vi "Main.vi"() -> ()   [LabVIEW 2014, in "DB_CONNECTOR.lvlib"]
doc: "Database Connector DQMH module. \n\nThis module is a singleton. Every module or component within an application that needs database connectivity should load its own instance of this module and keep the reference private.\n\n_____\nBased on Delacor QMH Project Template 4.0.0.43.\n\n<b>Note:</b> This VI was modified by the <b>Validate DQMH Module</b> tool to upgrade it to the DQMH 5.0 approach to destroying cloneable module event references.\n\n<b>Note:</b> This VI was modified by the <b>Validate DQMH Module</b> tool to have the module name be passed as the Additional Information parameter with an Error Reported broadcast.\n\n<b>Note:</b> This VI was modified by the <b>Validate DQMH Module</b> tool to call the Release Message Queue VI in the top-level Error case."
uses:
  DB_CONNECTOR.lvlib
  <vilib>/Delacor/Delacor QMH/Libraries/Cloneable Module Admin_class/Delacor_lib_QMH_Cloneable Module Admin.lvclass
  Module Data--cluster.ctl
  DB-Interface/DB-Interface.lvclass
  DB-Interface/DB-MySQL/Network Config.ctl
  <vilib>/Delacor/Delacor QMH/Libraries/Message Queue_class/Delacor_lib_QMH_Message Queue.lvclass/Delacor_lib_QMH_Message Queue.ctl
  <vilib>/Delacor/Delacor QMH/Libraries/Cloneable Module Admin_class/Delacor_lib_QMH_Cloneable Module Admin.lvclass/Delacor_lib_QMH_Cloneable Module Admin.ctl
  Stop Argument--cluster.ctl
  <vilib>/Delacor/Delacor QMH/Libraries/Module Admin_class/Delacor_lib_QMH_Module Admin.lvclass/Delacor_lib_QMH_Module Admin.ctl
  Configure Argument--cluster.ctl
  Connect Argument--cluster.ctl
  Query Argument--cluster.ctl
  Query (Reply Payload)--cluster.ctl
  Fast Query Argument--cluster.ctl
  Close Connection Argument--cluster.ctl
  Start Transaction Argument--cluster.ctl
  Commit Transaction Argument--cluster.ctl
  Commit Transaction (Reply Payload)--cluster.ctl
  Get DB-Type Argument--cluster.ctl
  Get DB-Type (Reply Payload)--cluster.ctl
  <vilib>/Utility/miscctls.llb/LVPointTypeDef.ctl
  <vilib>/Delacor/Delacor QMH/Libraries/Message Queue_class/Delacor_lib_QMH_Enqueue Message (Single).vi
  <vilib>/Delacor/Delacor QMH/Libraries/Cloneable Module Admin_class/Delacor_lib_QMH_Get Module ID.vi
  <vilib>/Delacor/Delacor QMH/Libraries/Module Admin_class/Delacor_lib_QMH_Get External Launch.vi
  <vilib>/Utility/error.llb/Error Cluster From Error Code.vi
  <vilib>/ErrorRing/Error Ring.xnode
  <vilib>/Delacor/Delacor QMH/Libraries/Message Queue_class/Delacor_lib_QMH_Message Queue.lvclass
  DB-Interface/DB-MySQL/DB-MySQL.lvclass
panel:
  in  "Config Section":string
  in  "Call Chain":string[](array[string])
  out "Module Name":string
  in  "Simulate MHL Error":bool
  in  "Simulate EHL Error":bool
  out "error out":errorcluster
  in  "Module Admin":refnum<class "Delacor_lib_QMH_Cloneable Module Admin.lvclass">
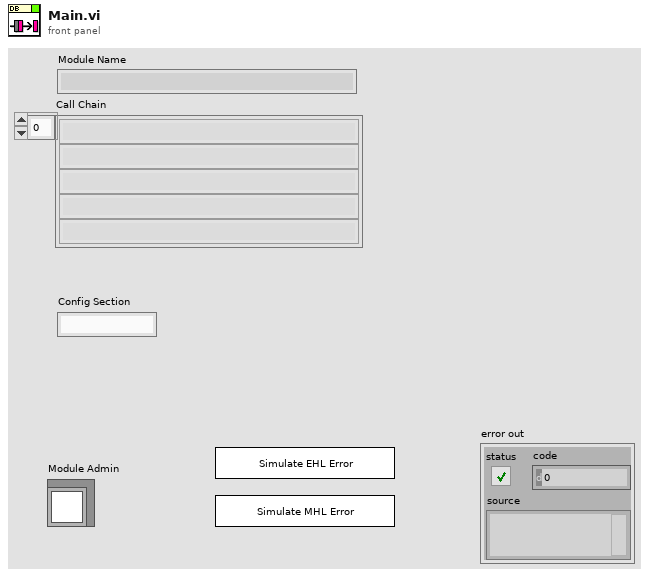
[diagram p1: front panel]
types:
  T1 = typedef "DB_CONNECTOR.lvlib/Request Events--cluster.ctl" = cluster{"Stop Module":refnum<user-event>, "Show Panel":refnum<user-event>, "Hide Panel":refnum<user-event>, "Show Diagram":refnum<user-event>, "Get Module Execution Status":refnum<user-event>, "Configure":refnum<user-event>, "Connect":refnum<user-event>, "Query":refnum<user-event>, "Close Connection":refnum<user-event>, "Start Transaction":refnum<user-event>, "Commit Transaction":refnum<user-event>, "Fast Query":refnum<user-event>, "Get DB-Type":refnum<user-event>}
  T2 = typedef "DB_CONNECTOR.lvlib/Module Data--cluster.ctl" = cluster{"Config Section":string, "DB-Interface":refnum<class "DB-Interface.lvclass">, "Driver":string, "DB-Type":string, "Authentication":cluster{"User":string, "Password":string, "Database":string}, "Network Config":T3}
  T3 = typedef "hse-db.lvlib/DB-MySQL.lvclass/Network Config.ctl" = cluster{"IP Address":string, "Port":u16, "Timeout ms":i32}
  T4 = enum32{"invalid lock state", "Not Locked", "Locked (No Password)", "Password-protected"}
  T5 = typedef "DB_CONNECTOR.lvlib/Stop Argument--cluster.ctl" = cluster{"Origin":string, "Module ID":i32, "Exit via Stop Module Req?":bool, "Wait for Module to stop?":bool}
  T6 = typedef "DB_CONNECTOR.lvlib/Configure Argument--cluster.ctl" = cluster{"Module ID":i32, "Boolean":bool}
  T7 = typedef "DB_CONNECTOR.lvlib/Connect Argument--cluster.ctl" = cluster{"Module ID":i32, "Boolean":bool}
  T8 = typedef "DB_CONNECTOR.lvlib/Query Argument--cluster.ctl" = cluster{"Module ID":i32, "Query":string, "Wait Notifier":refnum<notifier>}
  T9 = typedef "DB_CONNECTOR.lvlib/Fast Query Argument--cluster.ctl" = cluster{"Module ID":i32, "Query":string}
  T10 = typedef "DB_CONNECTOR.lvlib/Close Connection Argument--cluster.ctl" = cluster{"Module ID":i32, "Boolean":bool}
  T11 = typedef "DB_CONNECTOR.lvlib/Start Transaction Argument--cluster.ctl" = cluster{"Module ID":i32, "Boolean":bool}
  T12 = typedef "DB_CONNECTOR.lvlib/Commit Transaction Argument--cluster.ctl" = cluster{"Module ID":i32, "Wait Notifier":refnum<notifier>}
  T13 = typedef "DB_CONNECTOR.lvlib/Get DB-Type Argument--cluster.ctl" = cluster{"Module ID":i32, "Wait Notifier":refnum<notifier>, "wait for reply":bool}
  T14 = typedef "LVPointTypeDef.ctl" = cluster{"Horizontal":i16, "Vertical":i16}
  T15 = enum32{"Invalid", "Standard", "Closed", "Hidden", "Minimized", "Maximized"}
  T16 = typedef "DB_CONNECTOR.lvlib/Query (Reply Payload)--cluster.ctl" = cluster{"Return Data":string[][], "Meta Data":variant, "Field Names":string[], "Query_error":errorcluster}
  T17 = typedef "DB_CONNECTOR.lvlib/Commit Transaction (Reply Payload)--cluster.ctl" = cluster{"Commit Transaction_error":errorcluster}
  T18 = typedef "DB_CONNECTOR.lvlib/Get DB-Type (Reply Payload)--cluster.ctl" = cluster{"DB-Type":string, "error":errorcluster}
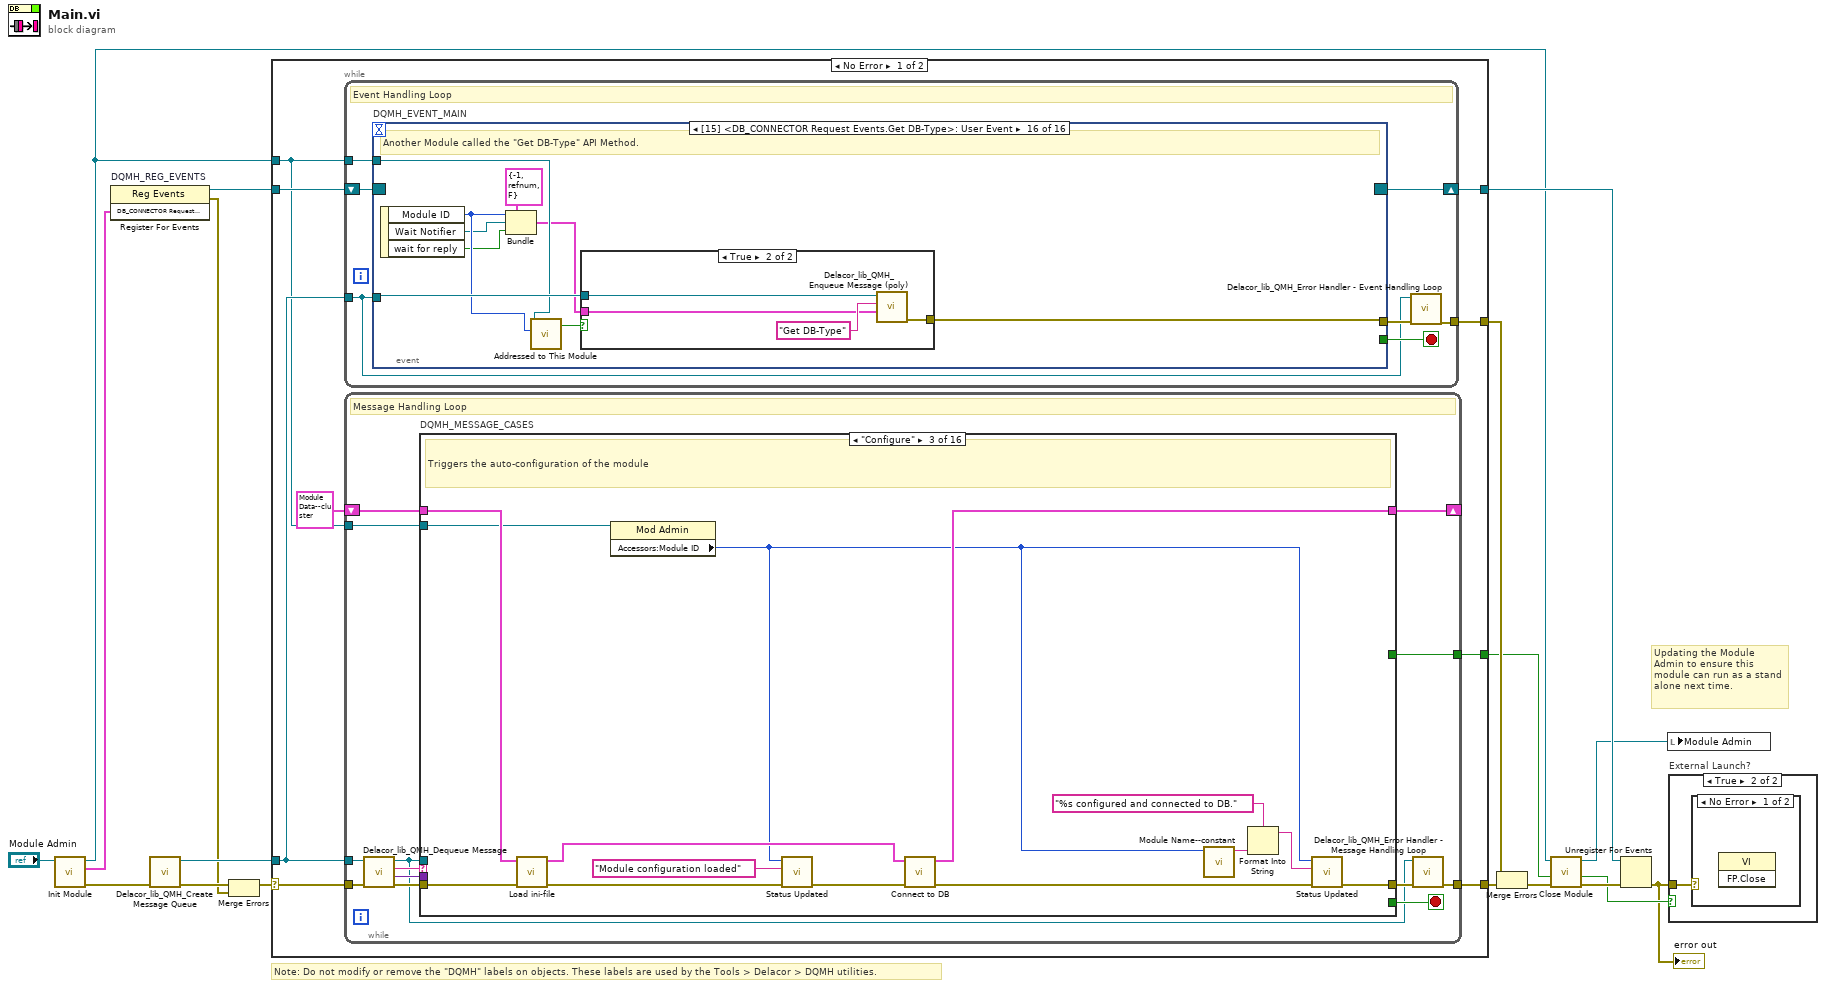
[diagram p0: block diagram]
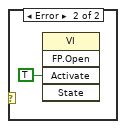
[diagram p3: hidden frame]
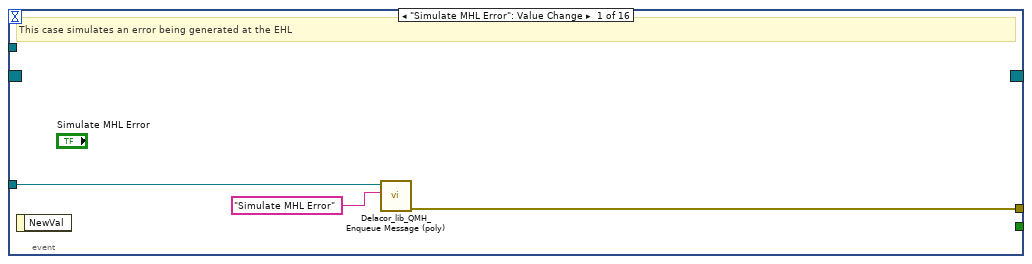
[diagram p4: hidden frame]
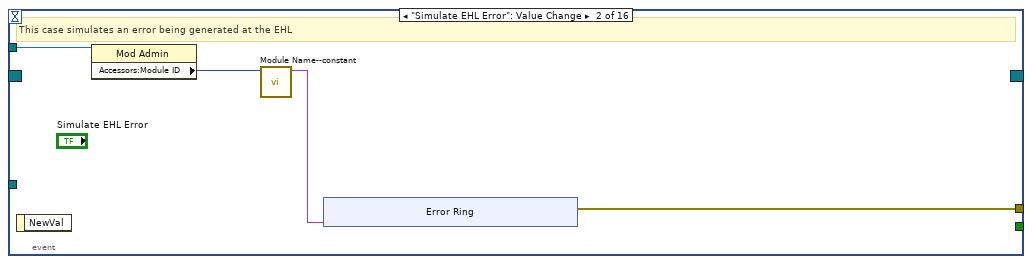
[diagram p5: hidden frame]
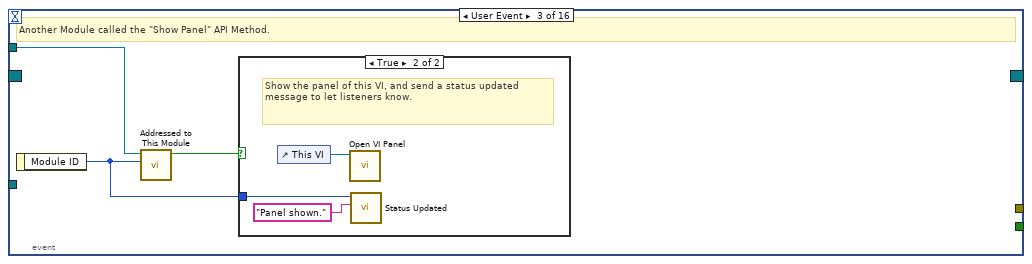
[diagram p6: hidden frame]
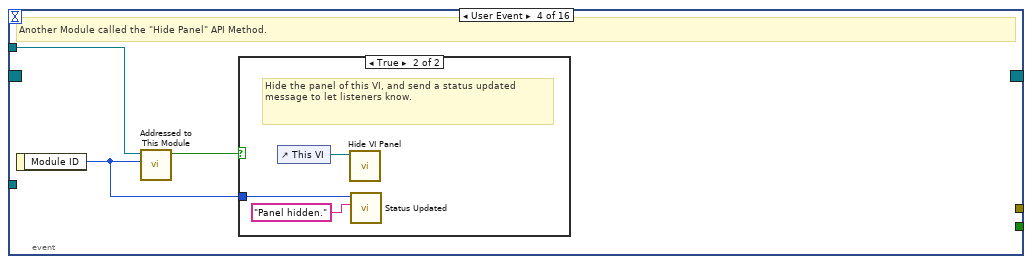
[diagram p8: hidden frame]
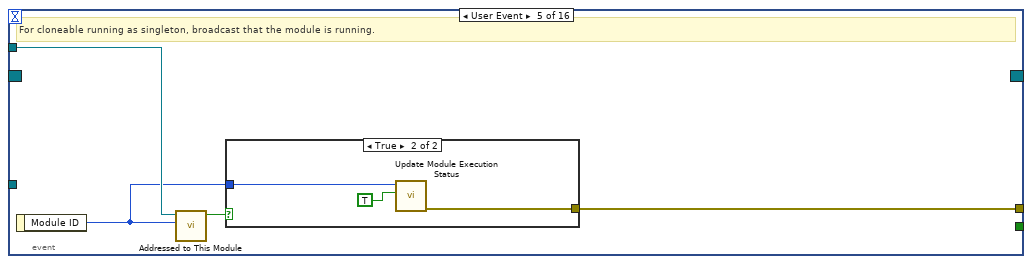
[diagram p10: hidden frame]
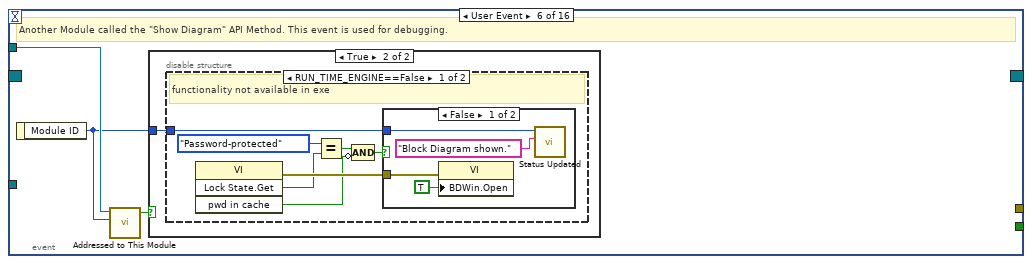
[diagram p12: hidden frame]
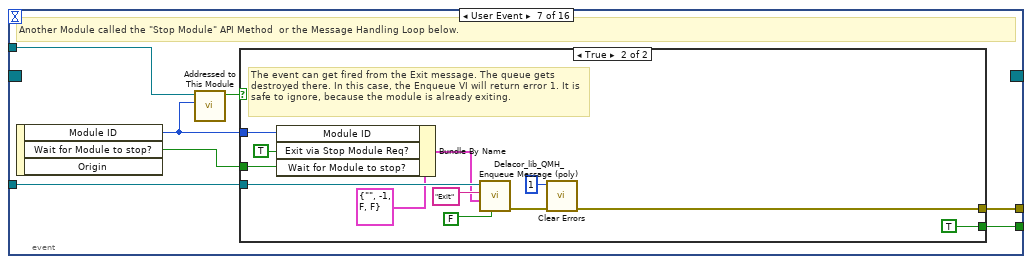
[diagram p16: hidden frame]
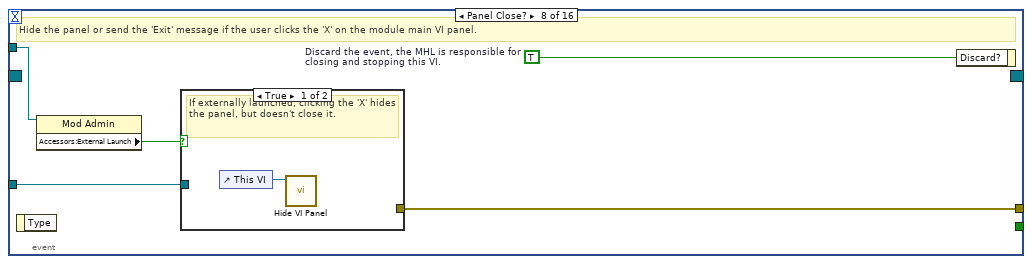
[diagram p18: hidden frame]
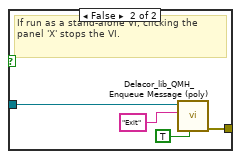
[diagram p19: hidden frame]
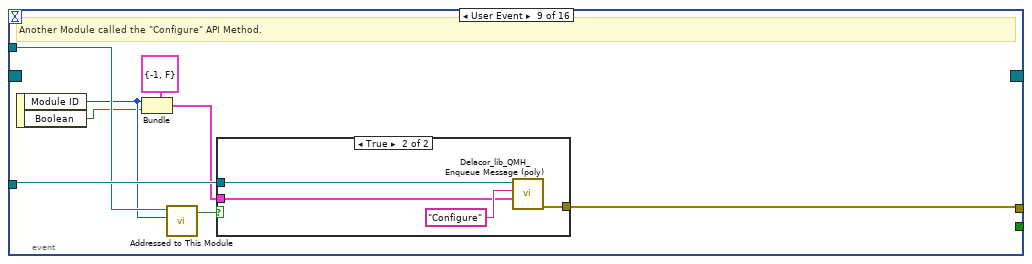
[diagram p20: hidden frame]
diagram:
  # "Note: Do not modify or remove the \"DQMH\" labels on objects. These labels are used by the Tools > Delacor > DQMH utilities."
  # "Updating the Module Admin to ensure this module can run as a stand alone next time."
  n1 = call "Init Module.vi"("Cloneable Module Admin in"="Module Admin") -> ("error out"=w15:errorcluster, "DB_CONNECTOR Request Events"=w12:T1, "Cloneable Module Admin out"=w8:refnum<class "Delacor_lib_QMH_Cloneable Module Admin.lvclass">)  [unwired: 8 in]
  n2 = register-events "DQMH_REG_EVENTS"(w12) -> (reference out=w13:refnum<event-registration>, error out=w3:errorcluster)  [unwired: 2 in]
  n3 = call <vilib>:"Delacor_lib_QMH_Create Message Queue.vi"("error in (no error)"=w15) -> ("error out"=w5:errorcluster, "Message Queue"=w11:refnum<class "Delacor_lib_QMH_Message Queue.lvclass">)  [unwired: 9 in]
  n4 = Merge Errors(w5, w3) -> (w4:errorcluster)
  n5 = case shown="No Error" w4 {
    selector: w4 -> [w21 w500]
    tunnel: [w27 w500] -> w16
    tunnel: [w26 w501] -> w14
    tunnel: w13 -> [w24 w501]
    tunnel: w11 -> [w23 w493]
    tunnel: [w22 _] -> w17
    tunnel: w8 -> [w20 w496]
    tunnel: [w19 _] -> w7
    frame No Error {
      n6 = while {
        tunnel: w23 -> [w28]
        shift-right: [w33] -> w26
        shift-left: w24 -> [w34]
        tunnel: [w30] -> w22
        tunnel: w20 -> [w29]
        stop <- w31 stop-if-true
        # "Event Handling Loop"
        n7 = event "DQMH_EVENT_MAIN" shown="[15] <DB_CONNECTOR Request Events.Get DB-Type>: User Event" {
          selector: w34 -> [_ _ _ _ _ _ _ _ _ _ _ _ _ _ _ _]
          dyn-events: [_ _ _ _ _ _ _ _ _ _ _ _ _ _ _ _] -> w33
          timeout: _ -> [_ _ _ _ _ _ _ _ _ _ _ _ _ _ _ _]
          tunnel: [_ _ _ _ _ _ w86 _ _ _ _ _ _ _ _ _] -> w31
          tunnel: w28 -> [w37 _ _ _ _ _ w89 w104 w119 w131 w144 w156 w168 w180 w192 w205]
          tunnel: [w36 w41 _ _ w62 _ w83 w102 w112 w124 w136 w149 w161 w173 w185 w197] -> w32
          tunnel: w29 -> [_ w40 w50 w56 w63 w69 w88 w105 w117 w129 w142 w154 w166 w178 w190 w203]
          event "Simulate MHL Error": Value Change {
            # "This case simulates an error being generated at the EHL"
            n8 = event-data() -> ()  [unwired: 1 in, 1 out]
            n9 = call-poly <vilib>:"Delacor_lib_QMH_Enqueue Message (poly).vi"("Message"="Simulate MHL Error", "Message Queue in"=w37) -> ("error out"=w36:errorcluster)  [unwired: 8 in, 1 out]
          }
          event "Simulate EHL Error": Value Change {
            # "This case simulates an error being generated at the EHL"
            n10 = event-data() -> ()  [unwired: 1 in, 1 out]
            n11 = property on="Property Node" class="Mod Admin"(reference=w40) -> ("Accessors:Module ID"=w39:i32)  [unwired: 1 in, 2 out]
            n12 = call "Module Name--constant.vi"("Module ID"=w39) -> ("Module Name"=w38:string)  [unwired: 10 in]
            n13 = xnode "Error Ring"("parameter 0"=w38) -> ("error out"=w41:errorcluster)
          }
          event User Event {
            # "Another Module called the \"Show Panel\" API Method."
            n14 = event-data() -> ("Module ID"=w49:i32)  [unwired: 1 in]
            n15 = call "Addressed to This Module.vi"("Module ID from Argument"=w49, "Module Admin"=w50) -> ("Addressed to this instance?"=w51:bool)  [unwired: 8 in, 1 out]
            n16 = case shown="True" w51 {
              tunnel: w49 -> [_ w52]
              frame False {
              }
              frame True {
                # "Show the panel of this VI, and send a status updated message to let listeners know."
                n17 = control-ref of="This VI"() -> (w54:refnum<vi>)
                n18 = call "Open VI Panel.vi"("VI"=w54) -> ()  [unwired: 10 in, 1 out]
                n19 = call "Status Updated.vi"("Status"="Panel shown." ("format string"), "Module ID"=w52) -> ()  [unwired: 9 in, 1 out]
              }
            }
          }
          event User Event {
            # "Another Module called the \"Hide Panel\" API Method."
            n20 = event-data() -> ("Module ID"=w55:i32)  [unwired: 1 in]
            n21 = call "Addressed to This Module.vi"("Module ID from Argument"=w55, "Module Admin"=w56) -> ("Addressed to this instance?"=w57:bool)  [unwired: 8 in, 1 out]
            n22 = case shown="True" w57 {
              tunnel: w55 -> [_ w58]
              frame False {
              }
              frame True {
                # "Hide the panel of this VI, and send a status updated message to let listeners know."
                n23 = control-ref of="This VI"() -> (w60:refnum<vi>)
                n24 = call "Hide VI Panel.vi"("VI"=w60) -> ()  [unwired: 10 in, 1 out]
                n25 = call "Status Updated.vi"("Status"="Panel hidden." ("format string"), "Module ID"=w58) -> ()  [unwired: 9 in, 1 out]
              }
            }
          }
          event User Event {
            # "For cloneable running as singleton, broadcast that the module is running."
            n26 = event-data() -> ("Module ID"=w61:i32)  [unwired: 1 in]
            n27 = call "Addressed to This Module.vi"("Module ID from Argument"=w61, "Module Admin"=w63) -> ("Addressed to this instance?"=w64:bool)  [unwired: 8 in, 1 out]
            n28 = case shown="True" w64 {
              tunnel: [_ w67] -> w62
              tunnel: w61 -> [_ w66]
              frame False {
              }
              frame True {
                n29 = call "Update Module Execution Status.vi"("Running?"=TRUE, "Module ID"=w66) -> ("error out"=w67:errorcluster)  [unwired: 9 in]
              }
            }
          }
          event User Event {
            # "Another Module called the \"Show Diagram\" API Method. This event is used for debugging."
            n30 = event-data() -> ("Module ID"=w68:i32)  [unwired: 1 in]
            n31 = call "Addressed to This Module.vi"("Module ID from Argument"=w68, "Module Admin"=w69) -> ("Addressed to this instance?"=w70:bool)  [unwired: 8 in, 1 out]
            n32 = case shown="True" w70 {
              tunnel: w68 -> [_ w71]
              frame False {
              }
              frame True {
                n33 = disable-structure shown="RUN_TIME_ENGINE==False" {
                  disable-tunnel: w71 -> [w72 _]
                  frame condition #0 (active) {
                    # "functionality not available in exe"
                    n34 = invoke on="Invoke Node" class="VI" method="Lock State.Get"() -> (error out=w78:errorcluster, "Get Lock State"=w77:T4, "pwd in cache"=w74:bool)  [unwired: 4 in, 1 out]
                    n35 = Equal?(x=T4."Password-protected", y=w77) -> (x = y?=w75:bool)
                    n36 = Compound Arithmetic op=AND(w75, invert w74) -> (w73:bool)
                    n37 = case shown="False" w73 {
                      tunnel: w78 -> [w81 _]
                      tunnel: w72 -> [w79 _]
                      frame False {
                        n38 = property on="Property Node" class="VI"(error in=w81, "BDWin.Open"=TRUE ("Block Diagram Window:Open")) -> ()  [unwired: 1 in, 2 out]
                        n39 = call "Status Updated.vi"("Status"="Block Diagram shown." ("format string"), "Module ID"=w79) -> ()  [unwired: 9 in, 1 out]
                      }
                      frame True {
                        # "Password-protected VI, and the password is not in the cache. Do not show the diagram."
                      }
                    }
                  }
                  frame condition #1 {
                  }
                }
              }
            }
          }
          event User Event {
            # "Another Module called the \"Stop Module\" API Method  or the Message Handling Loop below."
            n40 = event-data() -> ("Module ID"=w84:i32, "Wait for Module to stop?"=w85:bool)  [unwired: 1 in, 1 out]
            n41 = call "Addressed to This Module.vi"("Module ID from Argument"=w84, "Module Admin"=w88) -> ("Addressed to this instance?"=w87:bool)  [unwired: 8 in, 1 out]
            n42 = case shown="True" w87 {
              tunnel: [_ w91] -> w83
              tunnel: w89 -> [_ w97]
              tunnel: [_ TRUE] -> w86
              tunnel: w85 -> [_ w93]
              tunnel: w84 -> [_ w90]
              frame False {
              }
              frame True {
                # "The event can get fired from the Exit message. The queue gets destroyed there. In this case, the Enqueue VI will return error 1. It is safe to ignore, because the module is already exiting."
                n43 = Bundle By Name(cluster=T5 {"Origin"="", "Module ID"=-1, "Exit via Stop Module Req?"=FALSE, "Wait for Module to stop?"=FALSE} ("Stop Argument"), "Module ID"=w90, "Exit via Stop Module Req?"=TRUE, "Wait for Module to stop?"=w93) -> (w92:T5)
                n44 = call-poly <vilib>:"Delacor_lib_QMH_Enqueue Message (poly).vi"("Priority Message? (F)"=FALSE, "Message Data"=w92, "Message"="Exit", "Message Queue in"=w97) -> ("error out"=w100:errorcluster)  [unwired: 6 in, 1 out]
                n45 = call <vilib>:"Clear Errors.vi"("error in (no error)"=w100, "specific error code to clear (0: all)"=1) -> ("error out"=w91:errorcluster)  [unwired: 4 in, 1 out]
              }
            }
          }
          event Panel Close? {
            w106 = TRUE  # Discard the event, the MHL is responsible for closing and stopping this VI.
            # "Hide the panel or send the 'Exit' message if the user clicks the 'X' on the module main VI panel."
            n46 = event-data() -> ()  [unwired: 1 in, 1 out]
            n47 = property on="Property Node" class="Mod Admin"(reference=w105) -> ("Accessors:External Launch"=w103:bool)  [unwired: 1 in, 2 out]
            n48 = case shown="True" w103 {
              tunnel: w104 -> [_ w111]
              tunnel: [_ w110] -> w102
              frame True {
                # "If externally launched, clicking the 'X' hides the panel, but doesn't close it."
                n49 = control-ref of="This VI"() -> (w107:refnum<vi>)
                n50 = call "Hide VI Panel.vi"("VI"=w107) -> ()  [unwired: 10 in, 1 out]
              }
              frame False {
                # "If run as a stand-alone VI, clicking the panel 'X' stops the VI."
                n51 = call-poly <vilib>:"Delacor_lib_QMH_Enqueue Message (poly).vi"("Priority Message? (F)"=TRUE, "Message"="Exit", "Message Queue in"=w111) -> ("error out"=w110:errorcluster)  [unwired: 7 in, 1 out]
              }
            }
            n52 = event-data ("Event Filter Node")("Discard?"=w106) -> ()  [unwired: 1 in, 1 out]
          }
          event User Event {
            # "Another Module called the \"Configure\" API Method."
            n53 = event-data() -> ("Module ID"=w114:i32, "Boolean"=w113:bool)  [unwired: 1 in]
            n54 = Bundle(cluster=T6 {"Module ID"=-1, "Boolean"=FALSE} ("Configure Argument"), "Module ID"=w114, "Boolean"=w113) -> (w115:T6)
            n55 = call "Addressed to This Module.vi"("Module ID from Argument"=w114, "Module Admin"=w117) -> ("Addressed to this instance?"=w118:bool)  [unwired: 8 in, 1 out]
            n56 = case shown="True" w118 {
              tunnel: w119 -> [_ w123]
              tunnel: w115 -> [_ w121]
              tunnel: [_ w120] -> w112
              frame False {
              }
              frame True {
                n57 = call-poly <vilib>:"Delacor_lib_QMH_Enqueue Message (poly).vi"("Message Data"=w121, "Message"="Configure", "Message Queue in"=w123) -> ("error out"=w120:errorcluster)  [unwired: 7 in, 1 out]
              }
            }
          }
          event User Event {
            # "Another Module called the \"Connect\" API Method."
            n58 = event-data() -> ("Module ID"=w126:i32, "Boolean"=w125:bool)  [unwired: 1 in]
            n59 = Bundle(cluster=T7 {"Module ID"=-1, "Boolean"=FALSE} ("Connect Argument"), "Module ID"=w126, "Boolean"=w125) -> (w127:T7)
            n60 = call "Addressed to This Module.vi"("Module ID from Argument"=w126, "Module Admin"=w129) -> ("Addressed to this instance?"=w130:bool)  [unwired: 8 in, 1 out]
            n61 = case shown="True" w130 {
              tunnel: w131 -> [_ w135]
              tunnel: w127 -> [_ w133]
              tunnel: [_ w132] -> w124
              frame False {
              }
              frame True {
                n62 = call-poly <vilib>:"Delacor_lib_QMH_Enqueue Message (poly).vi"("Message Data"=w133, "Message"="Connect", "Message Queue in"=w135) -> ("error out"=w132:errorcluster)  [unwired: 7 in, 1 out]
              }
            }
          }
          event User Event {
            # "Another Module called the \"Query\" API Method."
            n63 = event-data() -> ("Module ID"=w139:i32, "Query"=w138:string, "Wait Notifier"=w137:refnum<notifier>)  [unwired: 1 in]
            n64 = Bundle(cluster=T8 {"Module ID"=-1, "Query"="", "Wait Notifier"=refnum} ("Query Argument"), "Module ID"=w139, "Query"=w138, "Wait Notifier"=w137) -> (w140:T8)
            n65 = call "Addressed to This Module.vi"("Module ID from Argument"=w139, "Module Admin"=w142) -> ("Addressed to this instance?"=w143:bool)  [unwired: 8 in, 1 out]
            n66 = case shown="True" w143 {
              tunnel: w144 -> [_ w148]
              tunnel: w140 -> [_ w146]
              tunnel: [_ w145] -> w136
              frame False {
              }
              frame True {
                n67 = call-poly <vilib>:"Delacor_lib_QMH_Enqueue Message (poly).vi"("Message Data"=w146, "Message"="Query", "Message Queue in"=w148) -> ("error out"=w145:errorcluster)  [unwired: 7 in, 1 out]
              }
            }
          }
          event User Event {
            # "Another Module called the \"Fast Query\" API Method."
            n68 = event-data() -> ("Module ID"=w151:i32, "Query"=w150:string)  [unwired: 1 in]
            n69 = Bundle(cluster=T9 {"Module ID"=-1, "Query"=""} ("Fast Query Argument"), "Module ID"=w151, "Query"=w150) -> (w152:T9)
            n70 = call "Addressed to This Module.vi"("Module ID from Argument"=w151, "Module Admin"=w154) -> ("Addressed to this instance?"=w155:bool)  [unwired: 8 in, 1 out]
            n71 = case shown="True" w155 {
              tunnel: w156 -> [_ w160]
              tunnel: w152 -> [_ w158]
              tunnel: [_ w157] -> w149
              frame False {
              }
              frame True {
                n72 = call-poly <vilib>:"Delacor_lib_QMH_Enqueue Message (poly).vi"("Message Data"=w158, "Message"="Fast Query", "Message Queue in"=w160) -> ("error out"=w157:errorcluster)  [unwired: 7 in, 1 out]
              }
            }
          }
          event User Event {
            # "Another Module called the \"Close Connection\" API Method."
            n73 = event-data() -> ("Module ID"=w163:i32, "Boolean"=w162:bool)  [unwired: 1 in]
            n74 = Bundle(cluster=T10 {"Module ID"=-1, "Boolean"=FALSE} ("Close Connection Argument"), "Module ID"=w163, "Boolean"=w162) -> (w164:T10)
            n75 = call "Addressed to This Module.vi"("Module ID from Argument"=w163, "Module Admin"=w166) -> ("Addressed to this instance?"=w167:bool)  [unwired: 8 in, 1 out]
            n76 = case shown="True" w167 {
              tunnel: w168 -> [_ w172]
              tunnel: w164 -> [_ w170]
              tunnel: [_ w169] -> w161
              frame False {
              }
              frame True {
                n77 = call-poly <vilib>:"Delacor_lib_QMH_Enqueue Message (poly).vi"("Message Data"=w170, "Message"="Close Connection", "Message Queue in"=w172) -> ("error out"=w169:errorcluster)  [unwired: 7 in, 1 out]
              }
            }
          }
          event User Event {
            # "Another Module called the \"Start Transaction\" API Method."
            n78 = event-data() -> ("Module ID"=w175:i32, "Boolean"=w174:bool)  [unwired: 1 in]
            n79 = Bundle(cluster=T11 {"Module ID"=-1, "Boolean"=FALSE} ("Start Transaction Argument"), "Module ID"=w175, "Boolean"=w174) -> (w176:T11)
            n80 = call "Addressed to This Module.vi"("Module ID from Argument"=w175, "Module Admin"=w178) -> ("Addressed to this instance?"=w179:bool)  [unwired: 8 in, 1 out]
            n81 = case shown="True" w179 {
              tunnel: w180 -> [_ w184]
              tunnel: w176 -> [_ w182]
              tunnel: [_ w181] -> w173
              frame False {
              }
              frame True {
                n82 = call-poly <vilib>:"Delacor_lib_QMH_Enqueue Message (poly).vi"("Message Data"=w182, "Message"="Start Transaction", "Message Queue in"=w184) -> ("error out"=w181:errorcluster)  [unwired: 7 in, 1 out]
              }
            }
          }
          event User Event {
            # "Another Module called the \"Commit Transaction\" API Method."
            n83 = event-data() -> ("Module ID"=w187:i32, "Wait Notifier"=w186:refnum<notifier>)  [unwired: 1 in]
            n84 = Bundle(cluster=T12 {"Module ID"=-1, "Wait Notifier"=refnum} ("Commit Transaction Argument"), "Module ID"=w187, "Wait Notifier"=w186) -> (w188:T12)
            n85 = call "Addressed to This Module.vi"("Module ID from Argument"=w187, "Module Admin"=w190) -> ("Addressed to this instance?"=w191:bool)  [unwired: 8 in, 1 out]
            n86 = case shown="True" w191 {
              tunnel: w192 -> [_ w196]
              tunnel: w188 -> [_ w194]
              tunnel: [_ w193] -> w185
              frame False {
              }
              frame True {
                n87 = call-poly <vilib>:"Delacor_lib_QMH_Enqueue Message (poly).vi"("Message Data"=w194, "Message"="Commit Transaction", "Message Queue in"=w196) -> ("error out"=w193:errorcluster)  [unwired: 7 in, 1 out]
              }
            }
          }
          event User Event {
            # "Another Module called the \"Get DB-Type\" API Method."
            n88 = event-data() -> ("Module ID"=w200:i32, "Wait Notifier"=w199:refnum<notifier>, "wait for reply"=w198:bool)  [unwired: 1 in]
            n89 = Bundle(cluster=T13 {"Module ID"=-1, "Wait Notifier"=refnum, "wait for reply"=FALSE} ("Get DB-Type Argument"), "Module ID"=w200, "Wait Notifier"=w199, "wait for reply"=w198) -> (w201:T13)
            n90 = call "Addressed to This Module.vi"("Module ID from Argument"=w200, "Module Admin"=w203) -> ("Addressed to this instance?"=w204:bool)  [unwired: 8 in, 1 out]
            n91 = case shown="True" w204 {
              tunnel: w205 -> [_ w209]
              tunnel: w201 -> [_ w207]
              tunnel: [_ w206] -> w197
              frame False {
              }
              frame True {
                n92 = call-poly <vilib>:"Delacor_lib_QMH_Enqueue Message (poly).vi"("Message Data"=w207, "Message"="Get DB-Type", "Message Queue in"=w209) -> ("error out"=w206:errorcluster)  [unwired: 7 in, 1 out]
              }
            }
          }
        }
        n93 = call-dynamic "Delacor_lib_QMH_Error Handler - Event Handling Loop.vi"("error in (no error)"=w32, "Message Queue in"=w28) -> ("dup error in"=w30:errorcluster)  [unwired: 8 in, 1 out]
      }
      n94 = while {
        tunnel: w23 -> [w214]
        shift-right: [w220] -> _
        shift-left: T2 {"Config Section"="", "DB-Interface"=refnum, "Driver"="", "DB-Type"="", "Authentication"={"User"="", "Password"="", "Database"=""}, "Network Config"={"IP Address"="", "Port"=0, "Timeout ms"=0}} ("Data Cluster") -> [w221]
        tunnel: w21 -> [w218]
        tunnel: [w212] -> w27
        tunnel: w20 -> [w211]
        tunnel: [w210] -> w19
        stop <- w219 stop-if-true
        # "Message Handling Loop"
        n95 = call-dynamic "Delacor_lib_QMH_Dequeue Message.vi"("error in (no error)"=w218, "Message Queue in"=w214) -> ("error out"=w217:errorcluster, "Message Data"=w215:variant, "Message"=w216:string, "Message Queue out"=w213:refnum<class "Delacor_lib_QMH_Message Queue.lvclass">)  [unwired: 6 in]
        n96 = case "DQMH_MESSAGE_CASES" shown="\"Configure\"" w216 {
          selector: w216 -> [_ _ _ _ _ _ _ _ _ _ _ _ _ _ _ w482]
          tunnel: w213 -> [_ _ _ _ _ _ _ _ _ _ _ _ w429 _ w475 _]
          tunnel: w217 -> [w242 w255 w269 w277 w282 w309 w362 w390 w407 w417 w424 w426 w438 w451 w476 w477]
          tunnel: [w225 w255 w258 w272 w278 w302 w341 w383 w401 w416 w422 w426 w428 w449 w462 w478] -> w222
          tunnel: w221 -> [w229 w254 w268 w276 w281 w299 w350 w381 w406 w410 w423 w425 w437 w450 w463 w484]
          tunnel: [w228 w254 w262 w275 w280 w298 w349 w380 w405 w410 w423 w425 w437 w450 w463 w484] -> w220
          tunnel: [_ _ _ _ _ _ _ _ _ _ _ _ _ _ w474 _] -> w219
          tunnel: w215 -> [_ _ _ _ _ w308 w360 w389 _ w415 _ _ w436 _ w469 _]
          tunnel: w211 -> [w238 _ w266 w274 _ w287 w345 _ w402 _ _ _ w433 w446 w465 w480]
          tunnel: [_ _ _ _ _ _ _ _ _ _ _ _ _ _ w467 _] -> w210
          frame "Initialize" {
            # "Initialize - Any operation that needs to be done before the module can receive messages. Synchronize Caller Events.vi will inform Start Module.vi that the module has launched and is ready to receive messages. Module Did Init.vi will broadcast that the module initialized."
            n97 = call "Synchronize Caller Events.vi"("error in (no error)"=w242, "Module Admin"=w238) -> ("error out"=w240:errorcluster, "Module Admin out"=w237:refnum<class "Delacor_lib_QMH_Cloneable Module Admin.lvclass">)  [unwired: 8 in]
            n98 = property on="Property Node" class="Mod Admin"(reference=w237) -> ("Accessors:Module ID"=w223:i32, "Accessors:External Launch"=w239:bool)  [unwired: 1 in, 2 out]
            n99 = call "Module Name--constant.vi"("Module ID"=w223) -> ("Module Name"=w243:string)  [unwired: 10 in]
            "Module Name" <- w243
            n100 = call "Module Name--constant.vi"("Module ID"=w223) -> ("Module Name"=w236:string)  [unwired: 10 in]
            n101 = disable-structure shown="TARGET_TYPE==Windows||EMBEDDED_UI==TRUE" {
              disable-tunnel: w243 -> [w249 _]
              disable-tunnel: w239 -> [w245 _]
              frame condition #0 (active) {
                n102 = property on="Property Node" class="VI"("Front Panel.Title"=w249) -> (reference out=w252:refnum<vi>, error out=w253:errorcluster)  [unwired: 2 in]
                n103 = Select(t=T15."Hidden" ("State"), s=w245, f=T15."Standard" ("State")) -> (s? t:f=w246:T15)
                n104 = invoke on="Invoke Node" class="VI" method="FP.Open"(reference=w252, error in=w253, "State"=w246) -> (reference out=w251:refnum<vi>, error out=w250:errorcluster)  [unwired: 2 in, 3 out]
                n105 = invoke on="Invoke Node" class="VI" method="FP.Center"(reference=w251, error in=w250) -> ()  [unwired: 1 in, 3 out]
                n106 = property on="Pane" class="Pane"("Origin"=T14 {"Horizontal"=0, "Vertical"=0}) -> ()  [unwired: 2 in, 2 out]
              }
              frame condition #1 {
              }
            }
            n107 = call "Module Did Init.vi"("error in (no error)"=w240, "Initialized?"=TRUE, "Origin"=w236, "Module ID"=w223) -> ("error out"=w226:errorcluster)  [unwired: 7 in]
            n108 = Reverse 1D Array(array="Call Chain") -> (reversed array=w233:string[])
            n109 = Index Array(array=w233) -> (element=w232:string)  [unwired: 1 in]
            n110 = Bundle By Name(cluster=w229, "Config Section"="Config Section") -> (w228:T2)
            n111 = Match Pattern(string=w232, regular expression=".lvlib") -> (before substring=w230:string)  [unwired: 1 in, 3 out]
            n112 = Format Into String(format string="%s initialised from %s", w236, w230) -> (resulting string=w224:string)  [unwired: 2 in, 1 out]
            n113 = call "Status Updated.vi"("error in (no error)"=w226, "Status"=w224, "Module ID"=w223) -> ("error out"=w225:errorcluster)  [unwired: 8 in]
          }
          frame "--- Module Specific ---" {
            # "Separator -- The following cases handle messages specific to this Module."
          }
          frame "Configure" {
            # "Triggers the auto-configuration of the module"
            n114 = call "Load ini-file.vi"("error in"=w269, "Data Cluster in"=w268) -> ("error out"=w265:errorcluster, "Data Cluster out"=w263:T2)  [unwired: 8 in]
            n115 = property on="Property Node" class="Mod Admin"(reference=w266) -> ("Accessors:Module ID"=w256:i32)  [unwired: 1 in, 2 out]
            n116 = call "Status Updated.vi"("error in (no error)"=w265, "Status"="Module configuration loaded", "Module ID"=w256) -> ("error out"=w264:errorcluster)  [unwired: 8 in]
            n117 = call "Connect to DB.vi"("error in"=w264, "Data Cluster in"=w263) -> ("error out"=w259:errorcluster, "Data Cluster out"=w262:T2)  [unwired: 8 in]
            n118 = call "Module Name--constant.vi"("Module ID"=w256) -> ("Module Name"=w261:string)  [unwired: 10 in]
            n119 = Format Into String(format string="%s configured and connected to DB.", w261) -> (resulting string=w257:string)  [unwired: 2 in, 1 out]
            n120 = call "Status Updated.vi"("error in (no error)"=w259, "Status"=w257, "Module ID"=w256) -> ("error out"=w258:errorcluster)  [unwired: 8 in]
          }
          frame "Connect" {
            w270 = "Connected to DB"  # Status
            # "Connect to database."
            n121 = call "Connect to DB.vi"("error in"=w277, "Data Cluster in"=w276) -> ("error out"=w271:errorcluster, "Data Cluster out"=w275:T2)  [unwired: 8 in]
            n122 = property on="Property Node" class="Mod Admin"(reference=w274) -> ("Accessors:Module ID"=w273:i32)  [unwired: 1 in, 2 out]
            n123 = call "Status Updated.vi"("error in (no error)"=w271, "Status"=w270, "Module ID"=w273) -> ("error out"=w272:errorcluster)  [unwired: 8 in]
          }
          frame "Start Transaction" {
            # "Start a transaction to get sure all following SQL commands get executed or none."
            n124 = Unbundle By Name(w281) -> ("DB-Interface"=w283:refnum<class "DB-Interface.lvclass">)
            n125 = call-dynamic "Start Transaction.vi"("error in"=w282, "DB-Interface in"=w283) -> ("error out"=w278:errorcluster, "DB-Interface out"=w279:refnum<class "DB-Interface.lvclass">)  [unwired: 8 in]
            n126 = Bundle By Name(cluster=w281, "DB-Interface"=w279) -> (w280:T2)
          }
          frame "Query" {
            # "#debugging\nBC status or error"
            # "Send a SQL-Query to the database."
            n127 = Variant To Data(error in=w309, type=T8 {"Module ID"=-1, "Query"="", "Wait Notifier"=refnum} ("Query Argument"), Variant=w308) -> (data=w306:T8, error out=w296:errorcluster)
            n128 = property on="Property Node" class="Mod Admin"(reference=w287) -> ("Accessors:Module ID"=w286:i32)  [unwired: 1 in, 2 out]
            n129 = Unbundle By Name(w299) -> ("DB-Interface"=w301:refnum<class "DB-Interface.lvclass">)
            n130 = Unbundle By Name(w306) -> ("Query"=w284:string, "Wait Notifier"=w305:refnum<notifier>)
            n131 = call-dynamic "Query.vi"("Query"=w284, "DB-Engine in"=w301) -> ("error out"=w295:errorcluster, "Meta Data"=w292:variant, "Return Data"=w293:string[][], "DB-Engine out"=w294:refnum<class "DB-Interface.lvclass">, "Field Names"=w291:string[])  [unwired: 5 in]
            n132 = case shown="Error" w295 {
              selector: w295 -> [w318 _]
              tunnel: [w319 w326] -> w297
              tunnel: w294 -> [w319 w330]
              tunnel: [w318 w324] -> w285
              tunnel: w284 -> [_ w323]
              tunnel: w293 -> [w317 _]
              tunnel: w292 -> [w316 _]
              tunnel: w291 -> [w315 _]
              tunnel: [w317 w322] -> w290
              tunnel: [w316 w321] -> w289
              tunnel: [w315 w320] -> w288
              frame No Error {
                # "No Error."
              }
              frame Error {
                # "Timeout or connection closed. Try to\nreconnect and send the query again."
                n133 = call-dynamic "Close.vi"("DB-Engine in"=w330) -> ("error out"=w328:errorcluster, "DB-Engine out"=w329:refnum<class "DB-Interface.lvclass">)  [unwired: 9 in]
                n134 = call-dynamic "Connect.vi"("error in"=w328, "DB-Engine in"=w329) -> ("error out"=w325:errorcluster, "DB-Engine out"=w327:refnum<class "DB-Interface.lvclass">)  [unwired: 8 in]
                n135 = call-dynamic "Query.vi"("error in"=w325, "Query"=w323, "DB-Engine in"=w327) -> ("error out"=w324:errorcluster, "Meta Data"=w321:variant, "Return Data"=w322:string[][], "DB-Engine out"=w326:refnum<class "DB-Interface.lvclass">, "Field Names"=w320:string[])  [unwired: 4 in]
              }
            }
            n136 = case shown="Error" w285 {
              selector: w285 -> [_ w313]
              tunnel: w286 -> [w311 w314]
              tunnel: w284 -> [w310 w312]
              frame No Error {
                n137 = call "Status Updated.vi"("Status"=w310, "Module ID"=w311) -> ()  [unwired: 9 in, 1 out]
              }
              frame Error {
                n138 = call "Error Reported.vi"("Additional Information"=w312, "Error"=w313, "Module ID"=w314) -> ()  [unwired: 8 in, 1 out]
              }
            }
            n139 = flat-sequence {
              tunnel: w305 -> [w337]
              tunnel: [w337] -> w304
              tunnel: [w336] -> w303
              tunnel: w285 -> [w332]
              tunnel: [w332] -> w300
              tunnel: w290 -> [w334]
              tunnel: w289 -> [w333]
              tunnel: w288 -> [w331]
              tunnel: w304 -> [w339]
              tunnel: w303 -> [w338]
              frame #0 {
                n140 = Bundle By Name(cluster=T16 {"Return Data"=[], "Meta Data"=variant(cluster{"Affected Rows":u64, "Insert ID":u64, "Server Status":u16, "Warning Count":u16, "Message":string} {"Affected Rows"=0, "Insert ID"=0, "Server Status"=0, "Warning Count"=0, "Message"=""}), "Field Names"=[], "Query_error"={"status"=FALSE, "code"=0, "source"=""}} ("Query (Reply Payload)"), "Return Data"=w334, "Meta Data"=w333, "Field Names"=w331, "Query_error"=w332) -> (w336:T16)
              }
              frame #1 {
                n141 = Send Notification(notification=w338, notifier=w339) -> ()  [unwired: 1 in, 2 out]
              }
            }
            n142 = Merge Errors(w296, w300) -> (w302:errorcluster)
            n143 = Bundle By Name(cluster=w299, "DB-Interface"=w297) -> (w298:T2)
          }
          frame "Fast Query" {
            # "An asynchonous query to the DB. This request does not block and has no reply. To receive the db response register to the corresponding broadcast."
            n144 = Variant To Data(error in=w362, type=T9 {"Module ID"=-1, "Query"=""} ("Fast Query Argument"), Variant=w360) -> (data=w358:T9, error out=w361:errorcluster)
            n145 = Unbundle By Name(w350) -> ("DB-Interface"=w352:refnum<class "DB-Interface.lvclass">)
            n146 = property on="Property Node" class="Mod Admin"(reference=w345) -> ("Accessors:Module ID"=w344:i32)  [unwired: 1 in, 2 out]
            n147 = Unbundle By Name(w358) -> ("Query"=w351:string)
            n148 = call-dynamic "Query.vi"("Query"=w351, "DB-Engine in"=w352) -> ("error out"=w357:errorcluster, "Meta Data"=w354:variant, "Return Data"=w355:string[][], "DB-Engine out"=w356:refnum<class "DB-Interface.lvclass">, "Field Names"=w353:string[])  [unwired: 5 in]
            n149 = case shown="No Error" w357 {
              selector: w357 -> [w366 _]
              tunnel: [w367 w374] -> w348
              tunnel: w356 -> [w367 w378]
              tunnel: [w366 w372] -> w347
              tunnel: w351 -> [_ w371]
              tunnel: w355 -> [w365 _]
              tunnel: w354 -> [w364 _]
              tunnel: w353 -> [w363 _]
              tunnel: [w365 w370] -> w346
              tunnel: [w364 w369] -> w343
              tunnel: [w363 w368] -> w342
              frame No Error {
                # "No Error."
              }
              frame Error {
                # "Timeout or connection closed. Try to\nreconnect and send the query again."
                n150 = call-dynamic "Close.vi"("DB-Engine in"=w378) -> ("error out"=w376:errorcluster, "DB-Engine out"=w377:refnum<class "DB-Interface.lvclass">)  [unwired: 9 in]
                n151 = call-dynamic "Connect.vi"("error in"=w376, "DB-Engine in"=w377) -> ("error out"=w373:errorcluster, "DB-Engine out"=w375:refnum<class "DB-Interface.lvclass">)  [unwired: 8 in]
                n152 = call-dynamic "Query.vi"("error in"=w373, "Query"=w371, "DB-Engine in"=w375) -> ("error out"=w372:errorcluster, "Meta Data"=w369:variant, "Return Data"=w370:string[][], "DB-Engine out"=w374:refnum<class "DB-Interface.lvclass">, "Field Names"=w368:string[])  [unwired: 4 in]
              }
            }
            n153 = call "Fast Query Reply.vi"("Field Names"=w342, "error in (no error)"=w347, "Meta Data"=w343, "Return Data"=w346, "Module ID"=w344) -> ("error out"=w340:errorcluster)  [unwired: 6 in]
            n154 = Bundle By Name(cluster=w350, "DB-Interface"=w348) -> (w349:T2)
            n155 = Merge Errors(w361, w340) -> (w341:errorcluster)
          }
          frame "Commit Transaction" {
            # "Commit a transaction. Either all SQL-commands get commited or, in case of an error, all get rejected."
            n156 = Variant To Data(error in=w390, type=T12 {"Module ID"=-1, "Wait Notifier"=refnum} ("Commit Transaction Argument"), Variant=w389) -> (data=w387:T12, error out=w391:errorcluster)
            n157 = Unbundle By Name(w387) -> ("Wait Notifier"=w386:refnum<notifier>)
            n158 = Unbundle By Name(w381) -> ("DB-Interface"=w382:refnum<class "DB-Interface.lvclass">)
            n159 = call-dynamic "Commit Transaction.vi"("error in"=w391, "DB-Interface in"=w382) -> ("error out"=w392:errorcluster, "DB-Interface out"=w379:refnum<class "DB-Interface.lvclass">)  [unwired: 8 in]
            n160 = Bundle By Name(cluster=w381, "DB-Interface"=w379) -> (w380:T2)
            n161 = flat-sequence {
              tunnel: w386 -> [w396]
              tunnel: [w396] -> w385
              tunnel: [w395] -> w384
              tunnel: w392 -> [w393]
              tunnel: w385 -> [w398]
              tunnel: w384 -> [w397]
              frame #0 {
                n162 = Bundle By Name(cluster=T17 {"Commit Transaction_error"={"status"=FALSE, "code"=0, "source"=""}} ("Commit Transaction (Reply Payload)"), "Commit Transaction_error"=w393) -> (w395:T17)
              }
              frame #1 {
                n163 = Send Notification(notification=w397, notifier=w398) -> ()  [unwired: 1 in, 2 out]
              }
            }
            n164 = Merge Errors(w391, w392) -> (w383:errorcluster)
          }
          frame "Close Connection" {
            # "Close connection to the database."
            n165 = Unbundle By Name(w406) -> ("DB-Interface"=w408:refnum<class "DB-Interface.lvclass">)
            n166 = call-dynamic "Close.vi"("error in"=w407, "DB-Engine in"=w408) -> ("error out"=w403:errorcluster, "DB-Engine out"=w404:refnum<class "DB-Interface.lvclass">)  [unwired: 8 in]
            n167 = Bundle By Name(cluster=w406, "DB-Interface"=w404) -> (w405:T2)
            n168 = property on="Property Node" class="Mod Admin"(reference=w402) -> ("Accessors:Module ID"=w400:i32)  [unwired: 1 in, 2 out]
            n169 = call "Status Updated.vi"("error in (no error)"=w403, "Status"="DB-connection closed", "Module ID"=w400) -> ("error out"=w401:errorcluster)  [unwired: 8 in]
          }
          frame "Get DB-Type" {
            # "Returns the type of the database in <b>DB-Type</b>"
            n170 = Variant To Data(error in=w417, type=T13 {"Module ID"=-1, "Wait Notifier"=refnum, "wait for reply"=FALSE} ("Get DB-Type Argument"), Variant=w415) -> (data=w413:T13, error out=w416:errorcluster)
            n171 = Unbundle By Name(w413) -> ("Wait Notifier"=w412:refnum<notifier>, "wait for reply"=w411:bool)
            n172 = Unbundle By Name(w410) -> ("DB-Type"=w409:string)
            n173 = case shown="True" w411 {
              tunnel: w412 -> [_ w421]
              tunnel: w409 -> [_ w420]
              frame False {
              }
              frame True {
                n174 = Bundle By Name(cluster=T18 {"DB-Type"="", "error"={"status"=FALSE, "code"=0, "source"=""}} ("Get DB-Type (Reply Payload)"), "DB-Type"=w420) -> (w418:T18)
                n175 = Send Notification(notification=w418, notifier=w421) -> ()  [unwired: 1 in, 2 out]
              }
            }
          }
          frame "---Copy This Frame---" {
            # "Duplicate this frame when creating new messages.  Change this comment in the duplicated frame to describe this message."
            n176 = Merge Errors(w424) -> (w422:errorcluster)
          }
          frame "--- Exit and Error Handling---" {
            # "Separator - the following cases handle errors and exit messages."
          }
          frame "Error" {
            # "Error - Check the error message data and respond accordingly. This message is sent by the \"Error Handler\" VIs at the end of each loop in this application."
            n177 = property on="Property Node" class="Mod Admin"(reference=w433) -> ("Accessors:External Launch"=w430:bool, "Accessors:Module ID"=w432:i32)  [unwired: 1 in, 2 out]
            n178 = Variant To Data(error in=w438, type=errorcluster {"status"=FALSE, "code"=0, "source"=""} ("error constant"), Variant=w436) -> (data=w439:errorcluster, error out=w434:errorcluster)
            n179 = call "Module Name--constant.vi"("Module ID"=w432) -> ("Module Name"=w427:string)  [unwired: 10 in]
            n180 = call "Error Reported.vi"("Additional Information"=w427, "Error"=w439, "Module ID"=w432) -> ()  [unwired: 8 in, 1 out]
            n181 = case shown="False" w430 {
              tunnel: [w444 _] -> w431
              tunnel: w429 -> [w443 _]
              tunnel: w439 -> [w440 _]
              frame False {
                # "If the module is running standalone, then pop up an error dialog and call the \"Exit\" message."
                n182 = call <vilib>:"Simple Error Handler.vi"("error in (no error)"=w440) -> ()  [unwired: 4 in, 5 out]
                n183 = call-poly <vilib>:"Delacor_lib_QMH_Enqueue Message (poly).vi"("Priority Message? (F)"=TRUE, "Message"="Exit", "Message Queue in"=w443) -> ("error out"=w444:errorcluster)  [unwired: 7 in, 1 out]
              }
              frame True {
                # "If the module was launched externally, calling the Error Reported broadcast VI is the only action performed by the \"Error\" message. The module's caller can then process the error appropriately."
              }
            }
            n184 = Merge Errors(w434, w431) -> (w428:errorcluster)
            n185 = local write "error out"(w428) -> ()
          }
          frame "Simulate MHL Error" {
            # "Simulate an error occurring at the MHL"
            n186 = property on="Property Node" class="Mod Admin"(reference=w446) -> ("Accessors:Module ID"=w447:i32)  [unwired: 1 in, 2 out]
            n187 = call "Module Name--constant.vi"("Module ID"=w447) -> ("Module Name"=w445:string)  [unwired: 10 in]
            n188 = xnode "Error Ring"("parameter 0"=w445) -> ("error out"=w448:errorcluster)
            n189 = Merge Errors(w451, w448) -> (w449:errorcluster)
          }
          frame "Exit" {
            w471 = 91  # 91: not all Exit messages will have an argument
            w474 = TRUE  # Stop the VI
            # "Release the message queue reference"
            # "Exit - Exit the application."
            n190 = Variant To Data(error in=w476, type=T5 {"Origin"="", "Module ID"=-1, "Exit via Stop Module Req?"=FALSE, "Wait for Module to stop?"=FALSE} ("Stop Argument"), Variant=w469) -> (data=w466:T5, error out=w470:errorcluster)
            n191 = call <vilib>:"Clear Errors.vi"("error in (no error)"=w470, "specific error code to clear (0: all)"=w471) -> ("error out"=w461:errorcluster)  [unwired: 4 in, 1 out]
            n192 = Unbundle By Name(w463) -> ("DB-Interface"=w459:refnum<class "DB-Interface.lvclass">)
            n193 = call-dynamic "Close.vi"("error in"=w461, "DB-Engine in"=w459) -> ("error out"=w460:errorcluster)  [unwired: 8 in, 1 out]
            n194 = control-ref of="This VI"() -> (w464:refnum<vi>)
            n195 = call-dynamic "Delacor_lib_QMH_Release Message Queue.vi"("error in (no error)"=w460, "Message Queue"=w475) -> ("error out"=w473:errorcluster)  [unwired: 9 in]
            n196 = call "Handle Exit.vi"("Stop Argument"=w466, "Module Admin in"=w465, "VI reference"=w464) -> ("error out"=w472:errorcluster, "Wait for Stop?"=w467:bool)  [unwired: 7 in]
            n197 = Merge Errors(w473, w472) -> (w462:errorcluster)
          }
          frame Default {
            # "'Default' case only runs if there is a message that isn't defined in any of the other cases.  Output a programming error."
            n198 = property on="Property Node" class="Mod Admin"(reference=w480) -> ("Accessors:Module ID"=w479:i32)  [unwired: 1 in, 2 out]
            n199 = call "Module Name--constant.vi"("Module ID"=w479) -> ("Module Name"=w481:string)  [unwired: 10 in]
            n200 = xnode "Error Ring"("parameter 0"=w482, "parameter 1"=w481) -> ("error out"=w483:errorcluster)
            n201 = Merge Errors(w477, w483) -> (w478:errorcluster)
          }
        }
        n202 = call-dynamic "Delacor_lib_QMH_Error Handler - Message Handling Loop.vi"("error in (no error)"=w222, "Message Queue in"=w213) -> ("dup error in"=w212:errorcluster)  [unwired: 8 in, 1 out]
      }
    }
    frame Error {
      n203 = call "Synchronize Caller Events.vi"("Module Admin"=w496) -> ("Module Admin out"=w495:refnum<class "Delacor_lib_QMH_Cloneable Module Admin.lvclass">)  [unwired: 9 in, 1 out]
      n204 = property on="Property Node" class="Mod Admin"(reference=w495) -> ("Accessors:Module ID"=w494:i32)  [unwired: 1 in, 2 out]
      n205 = call-dynamic "Delacor_lib_QMH_Release Message Queue.vi"("Message Queue"=w493) -> ()  [unwired: 10 in, 1 out]
      n206 = call "Module Name--constant.vi"("Module ID"=w494) -> ("Module Name"=w499:string)  [unwired: 10 in]
      n207 = Format Into String(format string="An error occurred during initialization. %s is no longer running.", w499) -> (resulting string=w497:string)  [unwired: 2 in, 1 out]
      n208 = call "Error Reported.vi"("Additional Information"=w497, "Error"=w500, "Module ID"=w494) -> ()  [unwired: 8 in, 1 out]
    }
  }
  n209 = Merge Errors(w17, w16) -> (w18:errorcluster)
  n210 = call "Close Module.vi"("error in (no error)"=w18, "Wait for stop?"=w7, "Module Admin in"=w8) -> ("error out"=w10:errorcluster, "External Launch"=w6:bool, "Module Admin out"=w1:refnum<class "Delacor_lib_QMH_Cloneable Module Admin.lvclass">)  [unwired: 6 in]
  n211 = Unregister For Events(event registration refnum=w14, error in=w10) -> (error out=w2:errorcluster)
  "error out" <- w2
  n212 = local write "Module Admin"(w1) -> ()
  n213 = case "External Launch?" shown="True" w6 {
    tunnel: w2 -> [_ w502]
    frame False {
    }
    frame True {
      n214 = case shown="No Error" w502 {
        frame No Error {
          n215 = invoke on="Invoke Node" class="VI" method="FP.Close"() -> ()  [unwired: 3 in, 3 out]
        }
        frame Error {
          n216 = invoke on="Invoke Node" class="VI" method="FP.Open"("Activate"=TRUE ("Activate?")) -> ()  [unwired: 4 in, 5 out]
        }
      }
    }
  }
